vi "testpath3.vi"() -> (4 "Trajectory":T1[](array[typedef])=[{"t"=0.0, "velocity"=0.0, "acceleration"=1.5000000000000002, "pose"={"Translation2d"={"x"=3.048, "y"=7.32}, "Rotation2d"={"Theta"=0.0}}, "curvature"=0.0}, {"t"=0.26318841870669524, "velocity"=0.39478262806004294, "acceleration"=1.4999999999999998, "pose"={"Translation2d"={"x"=3.099949943360352, "y"=7.319652167962023}, "Rotation2d"={"Theta"=-0.019971918166744478}}, "curvature"=-0.7636115223795371}, {"t"=0.36948492482788675, "velocity"=0.5542273872418302, "acceleration"=0.9893258261872959, "pose"={"Translation2d"={"x"=3.1503355546365754, "y"=7.317348982771782}, "Rotation2d"={"Theta"=-0.07810185233815051}}, "curvature"=-1.5647606140766166}, {"t"=0.4117570606819468, "velocity"=0.5960483029703497, "acceleration"=-1.3031431956514083, "pose"={"Translation2d"={"x"=3.1745290416453305, "y"=7.3149482814664}, "Rotation2d"={"Theta"=-0.12154551781557867}}, "curvature"=-2.018124199473524}, {"t"=0.4532301831920973, "velocity"=0.5420028855688298, "acceleration"=-1.0963837092013367, "pose"={"Translation2d"={"x"=3.1978728847629, "y"=7.311485558945839}, "Rotation2d"={"Theta"=-0.1749375579100152}}, "curvature"=-2.516292087881445}, {"t"=0.4973792029848024, "velocity"=0.4935986194909005, "acceleration"=-0.8959940799444455, "pose"={"Translation2d"={"x"=3.2202513084556, "y"=7.3068161003781}, "Rotation2d"={"Theta"=-0.2385314594754074}}, "curvature"=-3.0550678047878725}, {"t"=0.5442304458911938, "velocity"=0.4516201832087346, "acceleration"=-0.6977078164312602, "pose"={"Translation2d"={"x"=3.241565206302116, "y"=7.3008160266614945}, "Rotation2d"={"Theta"=-0.31235747491337007}}, "curvature"=-3.6158302060928915}, {"t"=0.59371280358814, "velocity"=0.4170959554681277, "acceleration"=-0.5502702892987111, "pose"={"Translation2d"={"x"=3.2617314998738003, "y"=7.2933814930504015}, "Rotation2d"={"Theta"=-0.3960059769552128}}, "curvature"=-4.161606365084675}, {"t"=0.6194191597231453, "velocity"=0.40295051144090266, "acceleration"=-0.4537944570015777, "pose"={"Translation2d"={"x"=3.2713625579263197, "y"=7.289099133232461}, "Rotation2d"={"Theta"=-0.4412109262460302}}, "curvature"=-4.412233912146192}, {"t"=0.6456792669078144, "velocity"=0.39103382036023254, "acceleration"=-0.35872337751457745, "pose"={"Translation2d"={"x"=3.280682497614963, "y"=7.284427887781026}, "Rotation2d"={"Theta"=-0.48841072855155615}}, "curvature"=-4.637444890788882}, {"t"=0.672427300998411, "velocity"=0.3814386752293787, "acceleration"=-0.26515659471242126, "pose"={"Translation2d"={"x"=3.289685156510468, "y"=7.279360053903572}, "Rotation2d"={"Theta"=-0.5373459655625523}}, "curvature"=-4.829008235209974}, {"t"=0.6995828713909455, "velocity"=0.3742381966566208, "acceleration"=-0.17306381081986122, "pose"={"Translation2d"={"x"=3.2983652537231674, "y"=7.273889030697156}, "Rotation2d"={"Theta"=-0.5877071696426507}}, "curvature"=-4.979214634058512}, {"t"=0.7270527510074084, "velocity"=0.3694841546074329, "acceleration"=-0.08230445614380336, "pose"={"Translation2d"={"x"=3.306718369868, "y"=7.268009294105475}, "Rotation2d"={"Theta"=-0.6391410543429558}}, "curvature"=-5.081595546929804}, {"t"=0.7547338372219726, "velocity"=0.36720587786107345, "acceleration"=0.007327002008865816, "pose"={"Translation2d"={"x"=3.3147409270295203, "y"=7.26171637187592}, "Rotation2d"={"Theta"=-0.6912605824921104}}, "curvature"=-5.1315991090878725}, {"t"=0.7825171548337527, "velocity"=0.3674094462850279, "acceleration"=0.09603775765468281, "pose"={"Translation2d"={"x"=3.322430168726906, "y"=7.2550068185166285}, "Rotation2d"={"Theta"=-0.7436582689510873}}, "curvature"=-5.12710596463869}, {"t"=0.810292539234296, "velocity"=0.37007693192085295, "acceleration"=0.1839647992565535, "pose"={"Translation2d"={"x"=3.329784139878969, "y"=7.247878190253543}, "Rotation2d"={"Theta"=-0.7959215893197124}}, "curvature"=-5.06868621850621}, {"t"=0.8379535169277367, "velocity"=0.37516557812946677, "acceleration"=0.2711047475886817, "pose"={"Translation2d"={"x"=3.3368016667691625, "y"=7.240329019987463}, "Rotation2d"={"Theta"=-0.8476489989740198}}, "curvature"=-4.959545409978163}, {"t"=0.8654018650808298, "velocity"=0.38260695562723734, "acceleration"=0.35725561353969615, "pose"={"Translation2d"={"x"=3.3434823370105917, "y"=7.2323587922511035}, "Rotation2d"={"Theta"=-0.8984649589344123}}, "curvature"=-4.805170257332568}, {"t"=0.8925513920592509, "velocity"=0.3923062765452257, "acceleration"=0.4419796232654606, "pose"={"Translation2d"={"x"=3.349826479511024, "y"=7.223967918166147}, "Rotation2d"={"Theta"=-0.9480325468739267}}, "curvature"=-4.612744537302747}, {"t"=0.9193306197316901, "velocity"=0.40414214950323035, "acceleration"=0.5245940453086011, "pose"={"Translation2d"={"x"=3.355835144437894, "y"=7.2151577104002955}, "Rotation2d"={"Theta"=-0.9960626519615907}}, "curvature"=-4.39044385259067}, {"t"=0.945684227977588, "velocity"=0.4179670954614241, "acceleration"=0.6041935808611568, "pose"={"Translation2d"={"x"=3.361510083183318, "y"=7.205930358124334}, "Rotation2d"={"Theta"=-1.0423192986977439}}, "curvature"=-4.146726130102364}, {"t"=0.9715732984686114, "velocity"=0.4336091056665624, "acceleration"=0.7153350615387603, "pose"={"Translation2d"={"x"=3.3668537283290987, "y"=7.1962889019691785}, "Rotation2d"={"Theta"=-1.0866211858450743}}, "curvature"=-3.889714967048319}, {"t"=1.0218188627011469, "velocity"=0.46955151944889295, "acceleration"=0.8424284702084108, "pose"={"Translation2d"={"x"=3.376560153887442, "y"=7.17577994758794}, "Rotation2d"={"Theta"=-1.1688959585687513}}, "curvature"=-3.364030064250997}, {"t"=1.0701152351915793, "velocity"=0.5102377586426234, "acceleration"=0.9380799882762356, "pose"={"Translation2d"={"x"=3.3849867442314645, "y"=7.153671249874651}, "Rotation2d"={"Theta"=-1.2424085833564584}}, "curvature"=-2.8583316258579563}, {"t"=1.116586221907962, "velocity"=0.553831261316713, "acceleration"=0.9976984170949652, "pose"={"Translation2d"={"x"=3.392175439275308, "y"=7.130015232061024}, "Rotation2d"={"Theta"=-1.307257225938115}}, "curvature"=-2.398952122349185}, {"t"=1.1614418998127427, "velocity"=0.5985837001600341, "acceleration"=1.0215095892207162, "pose"={"Translation2d"={"x"=3.3981771546090056, "y"=7.1048755366181675}, "Rotation2d"={"Theta"=-1.363907802949199}}, "curvature"=-1.9969630345874718}, {"t"=1.2049234360760661, "velocity"=0.6430005064070674, "acceleration"=1.0141956822707063, "pose"={"Translation2d"={"x"=3.4030511403787758, "y"=7.07832622388235}, "Rotation2d"={"Theta"=-1.4130182829288858}}, "curvature"=-1.6533172386850903}, {"t"=1.2472651193286828, "velocity"=0.6859432587419452, "acceleration"=0.9602009106383614, "pose"={"Translation2d"={"x"=3.406864340167318, "y"=7.050450970680747}, "Rotation2d"={"Theta"=-1.4553132146872148}}, "curvature"=-1.3633891597444852}, {"t"=1.3293491957534012, "velocity"=0.7647604636738685, "acceleration"=0.8586816816302829, "pose"={"Translation2d"={"x"=3.4116107765956682, "y"=6.99110062439801}, "Rotation2d"={"Theta"=-1.5222489468742204}}, "curvature"=-0.9159774788659977}, {"t"=1.4087890285949973, "velocity"=0.8329739929267188, "acceleration"=0.7675452912761603, "pose"={"Translation2d"={"x"=3.413081518736379, "y"=6.927655789984416}, "Rotation2d"={"Theta"=-1.5696286047023655}}, "curvature"=-0.5971075544889111}, {"t"=1.4860126079520202, "velocity"=0.8922465876376926, "acceleration"=0.7215507468236929, "pose"={"Translation2d"={"x"=3.41202368475422, "y"=6.861050335557494}, "Rotation2d"={"Theta"=-1.6010972924732694}}, "curvature"=-0.35962182913643914}, {"t"=1.5608683710367142, "velocity"=0.946258819395511, "acceleration"=0.7477618287923464, "pose"={"Translation2d"={"x"=3.4092459403057958, "y"=6.792295061162074}, "Rotation2d"={"Theta"=-1.6190734369903932}}, "curvature"=-0.16912085734671656}, {"t"=1.6327377531517113, "velocity"=0.9999999999999973, "acceleration"=-0.7477618287922758, "pose"={"Translation2d"={"x"=3.405597982708933, "y"=6.7224520547945215}, "Rotation2d"={"Theta"=-1.6249193382438716}}, "curvature"=-7.901475617054195e-15}, {"t"=1.7046071352667083, "velocity"=0.9462588193955163, "acceleration"=-0.7215507468237041, "pose"={"Translation2d"={"x"=3.40195002511207, "y"=6.652609048426969}, "Rotation2d"={"Theta"=-1.6190734369903943}}, "curvature"=0.16912085734669927}, {"t"=1.779462898351402, "velocity"=0.8922465876376973, "acceleration"=-0.7675452912761632, "pose"={"Translation2d"={"x"=3.3991722806636457, "y"=6.583853774031549}, "Rotation2d"={"Theta"=-1.6010972924732707}}, "curvature"=0.3596218291364221}, {"t"=1.8566864777084247, "velocity"=0.8329739929267235, "acceleration"=-0.8586816816302913, "pose"={"Translation2d"={"x"=3.398114446681486, "y"=6.517248319604627}, "Rotation2d"={"Theta"=-1.5696286047023693}}, "curvature"=0.5971075544888911}, {"t"=1.9361263105500202, "velocity"=0.764760463673873, "acceleration"=-0.9602009106384005, "pose"={"Translation2d"={"x"=3.399585188822197, "y"=6.453803485191033}, "Rotation2d"={"Theta"=-1.5222489468742246}}, "curvature"=0.9159774788659754}, {"t"=2.0182103869747365, "velocity"=0.6859432587419481, "acceleration"=-1.0141956822706626, "pose"={"Translation2d"={"x"=3.4043316252505473, "y"=6.394453138908297}, "Rotation2d"={"Theta"=-1.4553132146872205}}, "curvature"=1.3633891597444665}, {"t"=2.060552070227354, "velocity"=0.6430005064070712, "acceleration"=-1.0215095892206796, "pose"={"Translation2d"={"x"=3.408144825039089, "y"=6.366577885706693}, "Rotation2d"={"Theta"=-1.4130182829288918}}, "curvature"=1.6533172386850632}, {"t"=2.104033606490679, "velocity"=0.5985837001600383, "acceleration"=-0.9976984170950692, "pose"={"Translation2d"={"x"=3.4130188108088593, "y"=6.3400285729708745}, "Rotation2d"={"Theta"=-1.3639078029492069}}, "curvature"=1.9969630345874378}, {"t"=2.148889284395456, "velocity"=0.5538312613167158, "acceleration"=-0.9380799882762958, "pose"={"Translation2d"={"x"=3.4190205261425564, "y"=6.31488887752802}, "Rotation2d"={"Theta"=-1.307257225938124}}, "curvature"=2.3989521223491583}, {"t"=2.1953602711118387, "velocity"=0.5102377586426238, "acceleration"=-0.8424284702084165, "pose"={"Translation2d"={"x"=3.4262092211863995, "y"=6.291232859714393}, "Rotation2d"={"Theta"=-1.2424085833564666}}, "curvature"=2.8583316258579528}, {"t"=2.2436566436022707, "velocity"=0.4695515194488933, "acceleration"=-0.7153350615388038, "pose"={"Translation2d"={"x"=3.4346358115304216, "y"=6.269124162001104}, "Rotation2d"={"Theta"=-1.1688959585687604}}, "curvature"=3.364030064250993}, {"t"=2.2939022078348064, "velocity"=0.4336091056665604, "acceleration"=-0.6041935808611378, "pose"={"Translation2d"={"x"=3.444342237088765, "y"=6.248615207619865}, "Rotation2d"={"Theta"=-1.0866211858450845}}, "curvature"=3.889714967048351}, {"t"=2.3197912783258308, "velocity"=0.4179670954614221, "acceleration"=-0.5245940453086523, "pose"={"Translation2d"={"x"=3.4496858822345446, "y"=6.238973751464709}, "Rotation2d"={"Theta"=-1.0423192986977563}}, "curvature"=4.146726130102398}, {"t"=2.3461448865717274, "velocity"=0.40414214950322763, "acceleration"=-0.4419796232654363, "pose"={"Translation2d"={"x"=3.455360820979969, "y"=6.229746399188748}, "Rotation2d"={"Theta"=-0.9960626519616042}}, "curvature"=4.390443852590719}, {"t"=2.3729241142441673, "velocity"=0.3923062765452232, "acceleration"=-0.35725561353967616, "pose"={"Translation2d"={"x"=3.4613694859068396, "y"=6.220936191422897}, "Rotation2d"={"Theta"=-0.9480325468739386}}, "curvature"=4.612744537302796}, {"t"=2.4000736412225905, "velocity"=0.3826069556272347, "acceleration"=-0.27110474758883285, "pose"={"Translation2d"={"x"=3.467713628407272, "y"=6.2125453173379395}, "Rotation2d"={"Theta"=-0.8984649589344248}}, "curvature"=4.805170257332622}, {"t"=2.42752198937568, "velocity"=0.37516557812946094, "acceleration"=-0.18396479925663856, "pose"={"Translation2d"={"x"=3.4743942986486998, "y"=6.2045750896015806}, "Rotation2d"={"Theta"=-0.8476489989740319}}, "curvature"=4.959545409978286}, {"t"=2.45518296706912, "velocity"=0.3700769319208449, "acceleration"=-0.09603775765469771, "pose"={"Translation2d"={"x"=3.4814118255388937, "y"=6.197025919335502}, "Rotation2d"={"Theta"=-0.7959215893197208}}, "curvature"=5.068686218506383}, {"t"=2.482958351469662, "velocity"=0.3674094462850196, "acceleration"=-0.007327002008889338, "pose"={"Translation2d"={"x"=3.4887657966909558, "y"=6.189897291072416}, "Rotation2d"={"Theta"=-0.743658268951097}}, "curvature"=5.127105964638875}, {"t"=2.510741669081451, "velocity"=0.3672058778610644, "acceleration"=0.0823044561438033, "pose"={"Translation2d"={"x"=3.4964550383883424, "y"=6.183187737713124}, "Rotation2d"={"Theta"=-0.6912605824921165}}, "curvature"=5.1315991090880715}, {"t"=2.538422755296015, "velocity"=0.3694841546074238, "acceleration"=0.173063810819882, "pose"={"Translation2d"={"x"=3.5044775955498615, "y"=6.176894815483568}, "Rotation2d"={"Theta"=-0.6391410543429624}}, "curvature"=5.081595546930003}, {"t"=2.565892634912475, "velocity"=0.37423819665661173, "acceleration"=0.2651565947124028, "pose"={"Translation2d"={"x"=3.5128307116946935, "y"=6.171015078891888}, "Rotation2d"={"Theta"=-0.5877071696426573}}, "curvature"=4.979214634058704}, {"t"=2.5930482053050126, "velocity"=0.38143867522937003, "acceleration"=0.35872337751447186, "pose"={"Translation2d"={"x"=3.521510808907394, "y"=6.165544055685473}, "Rotation2d"={"Theta"=-0.5373459655625578}}, "curvature"=4.82900823521015}, {"t"=2.619796239395607, "velocity"=0.3910338203602203, "acceleration"=0.45379445700158316, "pose"={"Translation2d"={"x"=3.5305134678028973, "y"=6.160476221808018}, "Rotation2d"={"Theta"=-0.48841072855156026}}, "curvature"=4.637444890789121}, {"t"=2.6460563465802767, "velocity"=0.40295051144089095, "acceleration"=0.5502702892986385, "pose"={"Translation2d"={"x"=3.539833407491541, "y"=6.155804976356584}, "Rotation2d"={"Theta"=-0.4412109262460335}}, "curvature"=4.412233912146407}, {"t"=2.671762702715285, "velocity"=0.4170959554681157, "acceleration"=0.697707816431294, "pose"={"Translation2d"={"x"=3.5494644655440615, "y"=6.151522616538643}, "Rotation2d"={"Theta"=-0.3960059769552175}}, "curvature"=4.161606365084881}, {"t"=2.721245060412225, "velocity"=0.45162018320872005, "acceleration"=0.8959940799443867, "pose"={"Translation2d"={"x"=3.569630759115743, "y"=6.144088082927551}, "Rotation2d"={"Theta"=-0.31235747491337135}}, "curvature"=3.615830206093104}, {"t"=2.7680963033186217, "velocity"=0.4935986194908878, "acceleration"=1.096383709201355, "pose"={"Translation2d"={"x"=3.59094465696226, "y"=6.138088009210944}, "Rotation2d"={"Theta"=-0.2385314594754091}}, "curvature"=3.055067804788028}, {"t"=2.812245323111325, "velocity"=0.542002885568816, "acceleration"=1.3031431956514576, "pose"={"Translation2d"={"x"=3.6133230806549586, "y"=6.1334185506432055}, "Rotation2d"={"Theta"=-0.17493755791001384}}, "curvature"=2.516292087881585}, {"t"=2.853718445621474, "velocity"=0.5960483029703362, "acceleration"=1.4999999999999967, "pose"={"Translation2d"={"x"=3.636666923772527, "y"=6.129955828122645}, "Rotation2d"={"Theta"=-0.12154551781557543}}, "curvature"=2.0181241994736374}, {"t"=2.892604873611095, "velocity"=0.6543779449547675, "acceleration"=1.4999999999999962, "pose"={"Translation2d"={"x"=3.660860410781282, "y"=6.127555126817265}, "Rotation2d"={"Theta"=-0.0781018523381434}}, "curvature"=1.5647606140767099}, {"t"=2.963863246576663, "velocity"=0.7612655044031196, "acceleration"=1.0405196335401754, "pose"={"Translation2d"={"x"=3.711246022057505, "y"=6.125251941627026}, "Rotation2d"={"Theta"=-0.01997191816673276}}, "curvature"=0.763611522379592}, {"t"=3.029189820400926, "velocity"=0.8292390870591767, "acceleration"=-1.5, "pose"={"Translation2d"={"x"=3.7631959654178546, "y"=6.124904109589046}, "Rotation2d"={"Theta"=8.502859727842416e-15}}, "curvature"=1.0175126690166933e-14}, {"t"=3.0957507797886894, "velocity"=0.7293976479775318, "acceleration"=-1.5, "pose"={"Translation2d"={"x"=3.8150667797484186, "y"=6.125280265127143}, "Rotation2d"={"Theta"=0.02169629189301651}}, "curvature"=0.8370645436394706}, {"t"=3.169839919062551, "velocity"=0.6182639390667396, "acceleration"=-1.499999999999999, "pose"={"Translation2d"={"x"=3.8649281521524923, "y"=6.127770995623446}, "Rotation2d"={"Theta"=0.08595677451778284}}, "curvature"=1.782517383837334}, {"t"=3.2103029683127233, "velocity"=0.5575693651914811, "acceleration"=-1.4457439691216696, "pose"={"Translation2d"={"x"=3.8885749615894682, "y"=6.130367182842418}, "Rotation2d"={"Theta"=0.1350468581629947}}, "curvature"=2.362904642794918}, {"t"=3.25375724435825, "velocity"=0.49474560766611264, "acceleration"=-1.2078309552388122, "pose"={"Translation2d"={"x"=3.911130012707782, "y"=6.1341118702512905}, "Rotation2d"={"Theta"=0.1965838508185219}}, "curvature"=3.041081500714643}, {"t"=3.3007238350701016, "velocity"=0.43801790554230635, "acceleration"=-1.02600305040188, "pose"={"Translation2d"={"x"=3.932444367068773, "y"=6.139161556618315}, "Rotation2d"={"Theta"=0.2715148453026895}}, "curvature"=3.8205907799824077}, {"t"=3.3256552410396116, "velocity"=0.41243820696678135, "acceleration"=-0.9042303566046068, "pose"={"Translation2d"={"x"=3.9425956051051148, "y"=6.142218495388199}, "Rotation2d"={"Theta"=0.31423417016703553}}, "curvature"=4.242233471704546}, {"t"=3.351554605820681, "velocity"=0.3890192151149621, "acceleration"=-0.7827247383890393, "pose"={"Translation2d"={"x"=3.9523904547627575, "y"=6.14565020835563}, "Rotation2d"={"Theta"=0.3605071157677527}}, "curvature"=4.676881947505758}, {"t"=3.3784244404446717, "velocity"=0.36798753083834224, "acceleration"=-0.662602475512602, "pose"={"Translation2d"={"x"=3.9618161739669553, "y"=6.149470062822817}, "Rotation2d"={"Theta"=0.4102979234949962}}, "curvature"=5.114373635616514}, {"t"=3.4062447276670778, "velocity"=0.3495537396553043, "acceleration"=-0.544869386173178, "pose"={"Translation2d"={"x"=3.970861253571306, "y"=6.153690126148347}, "Rotation2d"={"Theta"=0.4634900930941465}}, "curvature"=5.541117727082771}, {"t"=3.434967334665074, "velocity"=0.33390367041101254, "acceleration"=-0.43022831997720556, "pose"={"Translation2d"={"x"=3.9795153917065753, "y"=6.158321192829343}, "Rotation2d"={"Theta"=0.5198699448216426}}, "curvature"=5.940400917104992}, {"t"=3.4645117522286055, "velocity"=0.32119282527794935, "acceleration"=-0.31896297108270455, "pose"={"Translation2d"={"x"=3.987769468129517, "y"=6.163372811583624}, "Rotation2d"={"Theta"=0.579114543882686}}, "curvature"=6.293329886337889}, {"t"=3.494763207006263, "velocity"=0.31154373138249364, "acceleration"=-0.21090669660756495, "pose"={"Translation2d"={"x"=3.995615518571693, "y"=6.168853312431866}, "Rotation2d"={"Theta"=0.6407871610915412}}, "curvature"=6.580475104760627}, {"t"=3.5255740996295852, "velocity"=0.30504550779977835, "acceleration"=-0.10549365407667427, "pose"={"Translation2d"={"x"=4.003046709088297, "y"=6.174769833779754}, "Rotation2d"={"Theta"=0.704343118936269}}, "curvature"=6.784090638880426}, {"t"=3.556769319971538, "velocity"=0.30175461001617876, "acceleration"=-0.00187984418221485, "pose"={"Translation2d"={"x"=4.010057310406972, "y"=6.181128349500149}, "Rotation2d"={"Theta"=0.7691476236098183}}, "curvature"=6.89055291686925}, {"t"=3.588155300244517, "velocity"=0.3016956092637595, "acceleration"=0.10088508839139915, "pose"={"Translation2d"={"x"=4.016642672276634, "y"=6.187933696015241}, "Rotation2d"={"Theta"=0.8345050811793373}}, "curvature"=6.892482815756199}, {"t"=3.619531844801653, "velocity"=0.30486103473482284, "acceleration"=0.2036584602787223, "pose"={"Translation2d"={"x"=4.022799197816295, "y"=6.195189599378709}, "Rotation2d"={"Theta"=0.8996969187800614}}, "curvature"=6.789997630017758}, {"t"=3.6507050870217803, "velocity"=0.3112097292472697, "acceleration"=0.3070031169576213, "pose"={"Translation2d"={"x"=4.028524317863877, "y"=6.202898702357883}, "Rotation2d"={"Theta"=0.964022866726053}}, "curvature"=6.590733441928565}, {"t"=3.6814996282233716, "velocity"=0.32066374938143816, "acceleration"=0.4110109916433966, "pose"={"Translation2d"={"x"=4.033816465325044, "y"=6.211062591515899}, "Rotation2d"={"Theta"=1.0268397706121166}}, "curvature"=6.308626742522132}, {"t"=3.711768130749851, "velocity"=0.3331044366204071, "acceleration"=0.5151787076413319, "pose"={"Translation2d"={"x"=4.038675049522012, "y"=6.219681824293856}, "Rotation2d"={"Theta"=1.087592646120109}}, "curvature"=5.96179886550171}, {"t"=3.7413972791782246, "velocity"=0.34836874301624976, "acceleration"=0.6183591380506606, "pose"={"Translation2d"={"x"=4.043100430542376, "y"=6.228755956092982}, "Rotation2d"={"Theta"=1.1458346067318108}}, "curvature"=5.570095425836476}, {"t"=3.77030984430284, "velocity"=0.3662470918655407, "acceleration"=0.7188046863919453, "pose"={"Translation2d"={"x"=4.047093893587934, "y"=6.238283567356788}, "Rotation2d"={"Theta"=1.201234763455285}}, "curvature"=5.152828512098055}, {"t"=3.798463311036893, "velocity"=0.38648393569215755, "acceleration"=0.8143044023369251, "pose"={"Translation2d"={"x"=4.050657623323499, "y"=6.248262290653226}, "Rotation2d"={"Theta"=1.2535754049779992}}, "curvature"=4.727095765043343}, {"t"=3.8258459843159427, "velocity"=0.40878176709104125, "acceleration"=0.9023998533373291, "pose"={"Translation2d"={"x"=4.053794678225729, "y"=6.25868883775685}, "Rotation2d"={"Theta"=1.3027411728436462}}, "curvature"=4.30681494355726}, {"t"=3.8524716267039065, "velocity"=0.43280874287695215, "acceleration"=0.9806482024487537, "pose"={"Translation2d"={"x"=4.056508964931945, "y"=6.269559026730973}, "Rotation2d"={"Theta"=1.3487034150678558}}, "curvature"=3.9024146353943783}, {"t"=3.8783735764649694, "velocity"=0.4582094433500563, "acceleration"=1.0737791801596355, "pose"={"Translation2d"={"x"=4.05880521258895, "y"=6.280867809009828}, "Rotation2d"={"Theta"=1.3915026250306526}}, "curvature"=3.5210103734247618}, {"t"=3.9281613757118374, "velocity"=0.511670545607311, "acceleration"=1.1493157053378875, "pose"={"Translation2d"={"x"=4.0621664659828935, "y"=6.304776788566211}, "Rotation2d"={"Theta"=1.468017807371216}}, "curvature"=2.841989124902466}, {"t"=3.9757359053738783, "velocity"=0.5663486997219579, "acceleration"=1.1670145631573443, "pose"={"Translation2d"={"x"=4.06393174702687, "y"=6.330359084440269}, "Rotation2d"={"Theta"=1.5333858309580786}}, "curvature"=2.2801144879387643}, {"t"=4.0215762991318815, "velocity"=0.6198451068184146, "acceleration"=1.1006743364612166, "pose"={"Translation2d"={"x"=4.06416588281649, "y"=6.357545871839132}, "Rotation2d"={"Theta"=1.588929308641928}}, "curvature"=1.8263218570407036}, {"t"=4.109815546037458, "velocity"=0.7169677813560476, "acceleration"=0.9318625883402352, "pose"={"Translation2d"={"x"=4.0603526943702315, "y"=6.4164021577786094}, "Rotation2d"={"Theta"=1.675700032982171}}, "curvature"=1.1755365710921948}, {"t"=4.195430482937836, "velocity"=0.79674913805662, "acceleration"=0.7523290288742276, "pose"={"Translation2d"={"x"=4.05144469510141, "y"=6.480585323804046}, "Rotation2d"={"Theta"=1.737246271947655}}, "curvature"=0.7596450332214446}, {"t"=4.279755261190648, "velocity"=0.8601891165895926, "acceleration"=0.6143533949739849, "pose"={"Translation2d"={"x"=4.038291441473745, "y"=6.549196386681844}, "Rotation2d"={"Theta"=1.7799721406425593}}, "curvature"=0.4840017650067866}, {"t"=4.363161607728101, "velocity"=0.911430088747253, "acceleration"=0.5350736721146327, "pose"={"Translation2d"={"x"=4.021847985150234, "y"=6.621225434656013}, "Rotation2d"={"Theta"=1.8081197219754728}}, "curvature"=0.2893761649681477}, {"t"=4.445300886137392, "velocity"=0.9553806540705587, "acceleration"=0.5216342862430297, "pose"={"Translation2d"={"x"=4.003148606186002, "y"=6.69557935957876}, "Rotation2d"={"Theta"=1.8243223962345434}}, "curvature"=0.1390742305568728}, {"t"=4.525300854255131, "velocity"=0.9971113803391205, "acceleration"=-0.4536998073169741, "pose"={"Translation2d"={"x"=3.9832805462211565, "y"=6.771109589041096}, "Rotation2d"={"Theta"=1.8300183745307899}}, "curvature"=0.00862673780876401}, {"t"=4.605089090371286, "velocity"=0.9609114729870597, "acceleration"=-0.5365543906927763, "pose"={"Translation2d"={"x"=3.9633577416736303, "y"=6.846639818503432}, "Rotation2d"={"Theta"=1.8256865496810237}}, "curvature"=-0.12113393775215417}, {"t"=4.686782126161709, "velocity"=0.9170787159446863, "acceleration"=-0.6130323265414291, "pose"={"Translation2d"={"x"=3.9444945569320353, "y"=6.9209937434261795}, "Rotation2d"={"Theta"=1.8109242098580547}}, "curvature"=-0.2692522327535906}, {"t"=4.769709532055165, "velocity"=0.8662415353757755, "acceleration"=-0.7505687846392907, "pose"={"Translation2d"={"x"=3.927779517548515, "y"=6.993022791400348}, "Rotation2d"={"Theta"=1.7843770627090099}}, "curvature"=-0.45981398932552625}, {"t"=4.853480716504348, "velocity"=0.8033654992759588, "acceleration"=-0.9338371634647636, "pose"={"Translation2d"={"x"=3.9142490434315893, "y"=7.061633854278146}, "Rotation2d"={"Theta"=1.7435098835081497}}, "curvature"=-0.7288639189517633}, {"t"=4.938416516388425, "velocity"=0.7240492928356015, "acceleration"=-1.1128693674812653, "pose"={"Translation2d"={"x"=3.9048611820390096, "y"=7.125817020303582}, "Rotation2d"={"Theta"=1.6841931776688028}}, "curvature"=-1.1349148706994323}, {"t"=5.025798137602182, "velocity"=0.6268049633059594, "acceleration"=-1.1909833664174907, "pose"={"Translation2d"={"x"=3.900469341570604, "y"=7.184673306243059}, "Rotation2d"={"Theta"=1.600125971053358}}, "curvature"=-1.7729779784640636}, {"t"=5.0711237586504465, "velocity"=0.5728229025649334, "acceleration"=-1.1815955171284798, "pose"={"Translation2d"={"x"=3.900378542851255, "y"=7.211860093641923}, "Rotation2d"={"Theta"=1.5461204056689204}}, "curvature"=-2.220687744773954}, {"t"=5.118131359885848, "velocity"=0.5172789316742191, "acceleration"=-1.1128857445929383, "pose"={"Translation2d"={"x"=3.901796024161135, "y"=7.237442389515981}, "Rotation2d"={"Theta"=1.4823867426308168}}, "curvature"=-2.7788901065523715}, {"t"=5.167314501619449, "velocity"=0.46254371436460084, "acceleration"=-0.9853196967791875, "pose"={"Translation2d"={"x"=3.9047873347963726, "y"=7.261351369072363}, "Rotation2d"={"Theta"=1.4075396162447975}}, "curvature"=-3.4601129169826157}, {"t"=5.219155935278846, "velocity"=0.41146332867072566, "acceleration"=-0.8579361355402367, "pose"={"Translation2d"={"x"=3.9094065590731395, "y"=7.283530340325342}, "Rotation2d"={"Theta"=1.3203628208481204}}, "curvature"=-4.259339937185443}, {"t"=5.24624506210542, "velocity"=0.3882225878859752, "acceleration"=-0.7617675977105636, "pose"={"Translation2d"={"x"=3.912340203217406, "y"=7.293956887428966}, "Rotation2d"={"Theta"=1.2719031149667976}}, "curvature"=-4.6925893076690235}, {"t"=5.274125426904337, "velocity"=0.36698422936981007, "acceleration"=-0.6600149113578105, "pose"={"Translation2d"={"x"=3.915695495489917, "y"=7.303935610725403}, "Rotation2d"={"Theta"=1.2201732587521121}}, "curvature"=-5.136496983697817}, {"t"=5.302795200406767, "velocity"=0.3480617513529555, "acceleration"=-0.5551081415780252, "pose"={"Translation2d"={"x"=3.919475606375281, "y"=7.31346322198921}, "Rotation2d"={"Theta"=1.1652564437436912}}, "curvature"=-5.577634725546802}, {"t"=5.33222209949546, "velocity"=0.33172664008742736, "acceleration"=-0.449032030653943, "pose"={"Translation2d"={"x"=3.923682835889786, "y"=7.322537353788336}, "Rotation2d"={"Theta"=1.107337414512981}}, "curvature"=-5.998928803965122}, {"t"=5.36233855927511, "velocity"=0.31820338499646317, "acceleration"=-0.3431550910056521, "pose"={"Translation2d"={"x"=3.9283185879302205, "y"=7.331156586566293}, "Rotation2d"={"Theta"=1.046716215748132}}, "curvature"=-6.380430087945608}, {"t"=5.393039206588993, "velocity"=0.3076683015735352, "acceleration"=-0.23815674690757505, "pose"={"Translation2d"={"x"=3.9333833446226927, "y"=7.339320475724309}, "Rotation2d"={"Theta"=0.9838145805699728}}, "curvature"=-6.700872755577214}, {"t"=5.424181717947586, "velocity"=0.3002515023778406, "acceleration"=-0.13405431784570007, "pose"={"Translation2d"={"x"=3.9388766406714555, "y"=7.347029578703482}, "Rotation2d"={"Theta"=0.9191717247022226}}, "curvature"=-6.9399556399395745}, {"t"=5.4555917701745775, "velocity"=0.2960408492530534, "acceleration"=-0.030315741458309037, "pose"={"Translation2d"={"x"=3.944797037707727, "y"=7.35428548206695}, "Rotation2d"={"Theta"=0.8534274890518816}}, "curvature"=-7.081018454188822}, {"t"=5.487072081656566, "velocity"=0.2950865002691384, "acceleration"=0.07396602536212296, "pose"={"Translation2d"={"x"=3.951142098638508, "y"=7.361090828582042}, "Rotation2d"={"Theta"=0.7872929428384307}}, "curvature"=-7.113550107943131}, {"t"=5.518414645078499, "velocity"=0.29740478511011903, "acceleration"=0.17986505233896102, "pose"={"Translation2d"={"x"=3.957908361995406, "y"=7.367449344302436}, "Rotation2d"={"Theta"=0.7215112626164027}}, "curvature"=-7.034887306172089}, {"t"=5.549414452573213, "velocity"=0.3029805671076536, "acceleration"=0.288409203225415, "pose"={"Translation2d"={"x"=3.9650913162834547, "y"=7.373365865650326}, "Rotation2d"={"Theta"=0.656814093888202}}, "curvature"=-6.850622256624144}, {"t"=5.579882613827221, "velocity"=0.3117678652186653, "acceleration"=0.4003883683441281, "pose"={"Translation2d"={"x"=3.9726853743299397, "y"=7.378846366498566}, "Rotation2d"={"Theta"=0.5938797909916396}}, "curvature"=-6.573603519065585}, {"t"=5.609656930959911, "velocity"=0.3236891554739839, "acceleration"=0.5162087737657857, "pose"={"Translation2d"={"x"=3.9806838476332143, "y"=7.383897985252849}, "Rotation2d"={"Theta"=0.5332994383480224}}, "curvature"=-6.221829571535764}, {"t"=5.638608652780793, "velocity"=0.33863428829354947, "acceleration"=0.6358147702330265, "pose"={"Translation2d"={"x"=3.9890789207115187, "y"=7.388529051933843}, "Rotation2d"={"Theta"=0.4755545834394751}}, "curvature"=-5.815815946306666}, {"t"=5.666645024556614, "velocity"=0.35646022757236073, "acceleration"=0.7586938982961912, "pose"={"Translation2d"={"x"=3.9978616254518116, "y"=7.392749115259375}, "Rotation2d"={"Theta"=0.4210079262946777}}, "curvature"=-5.376061416802838}, {"t"=5.693708067282841, "velocity"=0.3769927929580783, "acceleration"=0.8839721704593035, "pose"={"Translation2d"={"x"=4.007021815458583, "y"=7.3965689697265615}, "Rotation2d"={"Theta"=0.36990573115036535}}, "curvature"=-4.9210744088842135}, {"t"=5.719770547259522, "velocity"=0.40003129995061737, "acceleration"=1.010595158151202, "pose"={"Translation2d"={"x"=4.016548140402675, "y"=7.4000006826939915}, "Rotation2d"={"Theta"=0.32238910169973845}}, "curvature"=-4.466162591352536}, {"t"=5.744830274468121, "velocity"=0.4253565389322175, "acceleration"=1.2018608892153573, "pose"={"Translation2d"={"x"=4.026428020370103, "y"=7.403057621463877}, "Rotation2d"={"Theta"=0.27851067991033035}}, "curvature"=-4.022955833028221}, {"t"=5.7919336221573525, "velocity"=0.48196821027101827, "acceleration"=1.455458010218352, "pose"={"Translation2d"={"x"=4.047191823887849, "y"=7.4081073078309005}, "Rotation2d"={"Theta"=0.2015502334025534}}, "curvature"=-3.200648092862073}, {"t"=5.835376810367199, "velocity"=0.5451979465404633, "acceleration"=1.500000000000012, "pose"={"Translation2d"={"x"=4.069187020258681, "y"=7.411851995239773}, "Rotation2d"={"Theta"=0.1383803127731085}}, "curvature"=-2.4840945065364326}, {"t"=5.875734741636085, "velocity"=0.6057348434437911, "acceleration"=1.4999999999999953, "pose"={"Translation2d"={"x"=4.0922660886968085, "y"=7.414448182458744}, "Rotation2d"={"Theta"=0.0880295645890188}}, "curvature"=-1.8713804756786312}, {"t"=5.9495120585780255, "velocity"=0.7164008188567023, "acceleration"=1.5000000000000033, "pose"={"Translation2d"={"x"=4.140974258442265, "y"=7.416938912955046}, "Rotation2d"={"Theta"=0.02220021162873243}}, "curvature"=-0.8766770741906679}, {"t"=6.015703779688769, "velocity"=0.815688400522817, "acceleration"=-1.411158753722337, "pose"={"Translation2d"={"x"=4.191678674351594, "y"=7.417315068493148}, "Rotation2d"={"Theta"=-4.348736071993605e-15}}, "curvature"=4.6297649204425944e-29}, {"t"=6.081632420221635, "velocity"=0.72265262231385, "acceleration"=-1.5, "pose"={"Translation2d"={"x"=4.242387725084967, "y"=7.416949816014125}, "Rotation2d"={"Theta"=-0.021551071408703826}}, "curvature"=-0.8506112665210034}, {"t"=6.154699751119267, "velocity"=0.6130516259674026, "acceleration"=-1.500000000000001, "pose"={"Translation2d"={"x"=4.291125926643832, "y"=7.414531280604673}, "Rotation2d"={"Theta"=-0.08540110372174131}}, "curvature"=-1.8127044897775162}, {"t"=6.194563863764197, "velocity"=0.5532554570000089, "acceleration"=-1.4742082201926978, "pose"={"Translation2d"={"x"=4.314235733500783, "y"=7.412010345189149}, "Rotation2d"={"Theta"=-0.13420095994761355}}, "curvature"=-2.404548044357114}, {"t"=6.237379696389456, "velocity"=0.49013600458945655, "acceleration"=-1.2297545468345767, "pose"={"Translation2d"={"x"=4.336274624928279, "y"=7.408374199444301}, "Rotation2d"={"Theta"=-0.19540776415030497}}, "curvature"=-3.0976878160366175}, {"t"=6.283717050284497, "velocity"=0.43315243294874783, "acceleration"=-1.0438639863352206, "pose"={"Translation2d"={"x"=4.357096446235751, "y"=7.403470880798062}, "Rotation2d"={"Theta"=-0.2699944269844921}}, "curvature"=-3.896955421473778}, {"t"=6.3083408507292775, "velocity"=0.4074485344577359, "acceleration"=-0.9198414890264246, "pose"={"Translation2d"={"x"=4.367011030837094, "y"=7.400502548949043}, "Rotation2d"={"Theta"=-0.31254883046411347}}, "curvature"=-4.330651393103863}, {"t"=6.333939580128287, "velocity"=0.3839017610901667, "acceleration"=-0.7964221481695049, "pose"={"Translation2d"={"x"=4.376575985710204, "y"=7.397170305922697}, "Rotation2d"={"Theta"=-0.35867079037891914}}, "curvature"=-4.778920126845849}, {"t"=6.360517915374173, "velocity"=0.3627341862388689, "acceleration"=-0.6747263638224956, "pose"={"Translation2d"={"x"=4.385778799803259, "y"=7.393461171874849}, "Rotation2d"={"Theta"=-0.40833284223567334}}, "curvature"=-5.231570018449862}, {"t"=6.388058201331983, "velocity"=0.3441520292359239, "acceleration"=-0.5557590542485462, "pose"={"Translation2d"={"x"=4.394608170484017, "y"=7.389363429225421}, "Rotation2d"={"Theta"=-0.4614276486470032}}, "curvature"=-5.674828660300538}, {"t"=6.416514699519203, "velocity"=0.32833707271616924, "acceleration"=-0.44021373956923865, "pose"={"Translation2d"={"x"=4.403053978410674, "y"=7.384866596361266}, "Rotation2d"={"Theta"=-0.5177510355035748}}, "curvature"=-6.091599816339996}, {"t"=6.445809083367991, "velocity"=0.31544128245371733, "acceleration"=-0.32835366155801143, "pose"={"Translation2d"={"x"=4.411107262402737, "y"=7.379961401338992}, "Rotation2d"={"Theta"=-0.5769891409471082}}, "curvature"=-6.46237394112836}, {"t"=6.4758282443560695, "velocity"=0.3055843810263824, "acceleration"=-0.2199782815004123, "pose"={"Translation2d"={"x"=4.418760194311893, "y"=7.374639755587801}, "Rotation2d"={"Theta"=-0.6387129060337345}}, "curvature"=-6.766876284911729}, {"t"=6.506425405606849, "velocity"=0.29885367007564506, "acceleration"=-0.11447227589115234, "pose"={"Translation2d"={"x"=4.426006053892873, "y"=7.368894727612315}, "Rotation2d"={"Theta"=-0.7023828897284222}}, "curvature"=-6.986344232749775}, {"t"=6.537425160306578, "velocity"=0.29530505760309966, "acceleration"=-0.010924686245635714, "pose"={"Translation2d"={"x"=4.432839203674328, "y"=7.3627205166954095}, "Rotation2d"={"Theta"=-0.767366208906101}}, "curvature"=-7.106081407060201}, {"t"=6.568632368213271, "velocity"=0.2949641286481167, "acceleration"=0.09170049452982382, "pose"={"Translation2d"={"x"=4.43925506382969, "y"=7.356112426601046}, "Rotation2d"={"Theta"=-0.8329653207785563}}, "curvature"=-7.117736713801189}, {"t"=6.599844003444989, "velocity"=0.2978262510339498, "acceleration"=0.19436465441653678, "pose"={"Translation2d"={"x"=4.445250087048047, "y"=7.349066839277097}, "Rotation2d"={"Theta"=-0.8984558337431857}}, "curvature"=-7.020717906536788}, {"t"=6.630862316881653, "velocity"=0.3038551148056507, "acceleration"=0.29775030464725916, "pose"={"Translation2d"={"x"=4.450821733405006, "y"=7.341581188558189}, "Rotation2d"={"Theta"=-0.9631283452570845}}, "curvature"=-6.822334266969233}, {"t"=6.661507330894593, "velocity"=0.31297967706392316, "acceleration"=0.40207825036753225, "pose"={"Translation2d"={"x"=4.455968445233568, "y"=7.333653933868523}, "Rotation2d"={"Theta"=-1.0263282697065546}}, "curvature"=-6.536621755734763}, {"t"=6.691626862860313, "velocity"=0.3250900857785891, "acceleration"=0.5069727477723713, "pose"={"Translation2d"={"x"=4.460689621994987, "y"=7.32528453392471}, "Rotation2d"={"Theta"=-1.087488147579063}}, "curvature"=-6.182184923707348}, {"t"=6.721102904086689, "velocity"=0.3400336353925766, "acceleration"=0.611399064002761, "pose"={"Translation2d"={"x"=4.464985595149651, "y"=7.316473420438601}, "Rotation2d"={"Theta"=-1.1461488074139534}}, "curvature"=-5.77962728218252}, {"t"=6.749854018030981, "velocity"=0.35761203954715337, "acceleration"=0.7136909748896774, "pose"={"Translation2d"={"x"=4.46885760302794, "y"=7.307221971820122}, "Rotation2d"={"Theta"=-1.2019682666495493}}, "curvature"=-5.349154849994294}, {"t"=6.777834181656839, "velocity"=0.37758122980286485, "acceleration"=0.8116732069943011, "pose"={"Translation2d"={"x"=4.472307765701101, "y"=7.297532486880103}, "Rotation2d"={"Theta"=-1.254719563749324}}, "curvature"=-4.908764457929909}, {"t"=6.805028981536052, "velocity"=0.3996545202343935, "acceleration"=0.9028671117691384, "pose"={"Translation2d"={"x"=4.475339059852111, "y"=7.287408158533106}, "Rotation2d"={"Theta"=-1.3042802230553214}}, "curvature"=-4.473180516322608}, {"t"=6.831450240656345, "velocity"=0.423509406145637, "acceleration"=0.9847508747674881, "pose"={"Translation2d"={"x"=4.477955293646552, "y"=7.276853047500262}, "Rotation2d"={"Theta"=-1.3506165973360953}}, "curvature"=-4.053489703016462}, {"t"=6.857130057884056, "velocity"=0.4487976286244948, "acceleration"=1.0840978528150274, "pose"={"Translation2d"={"x"=4.480161081603476, "y"=7.265872056012099}, "Rotation2d"={"Theta"=-1.3937660908844118}}, "curvature"=-3.6572987095129776}, {"t"=6.906415424080401, "velocity"=0.5022277882931547, "acceleration"=1.1681738456180772, "pose"={"Translation2d"={"x"=4.48336365907354, "y"=7.242656090355901}, "Rotation2d"={"Theta"=-1.4709054934935915}}, "curvature"=-2.951411863769849}, {"t"=6.9534146874062905, "velocity"=0.5571310984737756, "acceleration"=1.193511382535945, "pose"={"Translation2d"={"x"=4.48499888057713, "y"=7.21781531030428}, "Rotation2d"={"Theta"=-1.5367982374777283}}, "curvature"=-2.3671059273267914}, {"t"=6.998610709889867, "velocity"=0.6110730657532749, "acceleration"=1.167228878425908, "pose"={"Translation2d"={"x"=4.48513012782019, "y"=7.191416545728572}, "Rotation2d"={"Theta"=-1.5927777102801355}}, "curvature"=-1.8952861433421067}, {"t"=7.0424478424442185, "velocity"=0.6622410328180989, "acceleration"=1.1031072318105943, "pose"={"Translation2d"={"x"=4.483831271767576, "y"=7.163537566122281}, "Rotation2d"={"Theta"=-1.6401769535401651}}, "curvature"=-1.5187654555632588}, {"t"=7.085299075903088, "velocity"=0.7095105383385827, "acceleration"=0.9684377738130721, "pose"={"Translation2d"={"x"=4.481185868510851, "y"=7.134266239091687}, "Rotation2d"={"Theta"=-1.680211297171634}}, "curvature"=-1.2191901359084476}, {"t"=7.169232040012571, "velocity"=0.790794391250303, "acceleration"=0.7862293281400811, "pose"={"Translation2d"={"x"=4.472233245591629, "y"=7.071943454690177}, "Rotation2d"={"Theta"=-1.7422278435917522}}, "curvature"=-0.7877885280324147}, {"t"=7.251717497665008, "velocity"=0.8556468772017057, "acceleration"=0.6443002943750661, "pose"={"Translation2d"={"x"=4.459103853305386, "y"=7.0053211182726045}, "Rotation2d"={"Theta"=-1.785308378900926}}, "curvature"=-0.5023790527257399}, {"t"=7.333169771733416, "velocity"=0.9081266013614995, "acceleration"=0.5623075046520477, "pose"={"Translation2d"={"x"=4.4427327834611825, "y"=6.935379868790441}, "Rotation2d"={"Theta"=-1.813745214747585}}, "curvature"=-0.3012612639388497}, {"t"=7.41328161180343, "velocity"=0.9531740902443532, "acceleration"=0.5488855969790963, "pose"={"Translation2d"={"x"=4.4241328932037085, "y"=6.863181130097338}, "Rotation2d"={"Theta"=-1.8302042982477884}}, "curvature"=-0.14628975216743031}, {"t"=7.491221325535914, "velocity"=0.9959540765447876, "acceleration"=-0.45125036796996526, "pose"={"Translation2d"={"x"=4.404369072782734, "y"=6.789840182648404}, "Rotation2d"={"Theta"=-1.8361458971072677}}, "curvature"=-0.012097016067171314}, {"t"=7.568872140041282, "velocity"=0.9609141179260725, "acceleration"=-0.5647024525910581, "pose"={"Translation2d"={"x"=4.384532513322541, "y"=6.716499235199469}, "Rotation2d"={"Theta"=-1.8320649407218288}}, "curvature"=0.12112540777990023}, {"t"=7.648374940406329, "velocity"=0.9160186915720734, "acceleration"=-0.6426968844949578, "pose"={"Translation2d"={"x"=4.365714974591368, "y"=6.644300496506366}, "Rotation2d"={"Theta"=-1.8175711668267878}}, "curvature"=0.27300978311453855}, {"t"=7.7291731327763475, "velocity"=0.8640899450630382, "acceleration"=-0.7840912084570016, "pose"={"Translation2d"={"x"=4.348983052770848, "y"=6.574359247024203}, "Rotation2d"={"Theta"=-1.7913197948653747}}, "curvature"=0.4683737482570857}, {"t"=7.810902047747827, "velocity"=0.8000070213571715, "acceleration"=-0.9717670823993614, "pose"={"Translation2d"={"x"=4.335352448225446, "y"=6.507736910606631}, "Rotation2d"={"Theta"=-1.750780406494041}}, "curvature"=0.7444248447082671}, {"t"=7.89390622691947, "velocity"=0.7193462923365892, "acceleration"=-1.1525167861686512, "pose"={"Translation2d"={"x"=4.325762233271908, "y"=6.4454141262051206}, "Rotation2d"={"Theta"=-1.6918170448995062}}, "curvature"=1.1618035078482665}, {"t"=7.979491291568851, "velocity"=0.6207080686828482, "acceleration"=-1.2279138106159257, "pose"={"Translation2d"={"x"=4.321049119948684, "y"=6.3882638195682375}, "Rotation2d"={"Theta"=-1.6080938154691222}}, "curvature"=1.819642710916439}, {"t"=8.023982023933382, "velocity"=0.5660772839680233, "acceleration"=-1.213987143459038, "pose"={"Translation2d"={"x"=4.32074862723075, "y"=6.361865054992528}, "Rotation2d"={"Theta"=-1.554229183834945}}, "curvature"=2.282635502335119}, {"t"=8.070204152701344, "velocity"=0.5099642139004098, "acceleration"=-1.1390484102972946, "pose"={"Translation2d"={"x"=4.321921727785386, "y"=6.337024274940908}, "Rotation2d"={"Theta"=-1.4905873873528683}}, "curvature"=2.8614621422727504}, {"t"=8.118660432929483, "velocity"=0.45477016493762756, "acceleration"=-1.0439844750065996, "pose"={"Translation2d"={"x"=4.32463276290521, "y"=6.31380830928471}, "Rotation2d"={"Theta"=-1.415749206631394}}, "curvature"=3.5701589836797614}, {"t"=8.143916319635684, "velocity"=0.42840341131382703, "acceleration"=-0.9632744975641985, "pose"={"Translation2d"={"x"=4.326582065968441, "y"=6.302827317796546}, "Rotation2d"={"Theta"=-1.3737223202829167}}, "curvature"=3.973165143670482}, {"t"=8.169919428646885, "velocity"=0.4033552795459559, "acceleration"=-0.8720074406733708, "pose"={"Translation2d"={"x"=4.3289348515722175, "y"=6.292272206763702}, "Rotation2d"={"Theta"=-1.328453402042927}}, "curvature"=4.404817963130555}, {"t"=8.19671230377379, "velocity"=0.3799916930782627, "acceleration"=-0.7728544180566954, "pose"={"Translation2d"={"x"=4.331695874175318, "y"=6.282147878416706}, "Rotation2d"={"Theta"=-1.2798699246501777}}, "curvature"=4.858736136815974}, {"t"=8.224319123226767, "velocity"=0.35865564069553557, "acceleration"=-0.6685443626921248, "pose"={"Translation2d"={"x"=4.334869086325574, "y"=6.272458393476687}, "Rotation2d"={"Theta"=-1.2279647766292976}}, "curvature"=5.324925338385862}, {"t"=8.252739248295114, "velocity"=0.3396555262940866, "acceleration"=-0.5615677589366793, "pose"={"Translation2d"={"x"=4.3384576135307515, "y"=6.263206944858208}, "Rotation2d"={"Theta"=-1.1728156577162963}}, "curvature"=5.789376201433284}, {"t"=8.281940952895548, "velocity"=0.3232567904844901, "acceleration"=-0.45392550811035604, "pose"={"Translation2d"={"x"=4.342463729129415, "y"=6.2543958313721}, "Rotation2d"={"Theta"=-1.1146035916342591}}, "curvature"=6.2341343733371914}, {"t"=8.311856306790474, "velocity"=0.3096774482674344, "acceleration"=-0.34696015155136106, "pose"={"Translation2d"={"x"=4.346888829161787, "y"=6.246026431428286}, "Rotation2d"={"Theta"=-1.0536275630080953}}, "curvature"=6.63807860036062}, {"t"=8.342378391588255, "velocity"=0.299087501100333, "acceleration"=-0.24128875012029047, "pose"={"Translation2d"={"x"=4.351733407240634, "y"=6.238099176738619}, "Rotation2d"={"Theta"=-0.9903117021356771}}, "curvature"=6.978554094160373}, {"t"=8.373362001111014, "velocity"=0.2916115046843714, "acceleration"=-0.13683731223853002, "pose"={"Translation2d"={"x"=4.356997029422121, "y"=6.230613526019712}, "Rotation2d"={"Theta"=-0.9252015770462301}}, "curvature"=7.233804284983293}, {"t"=8.404628601498835, "velocity"=0.2873330671244657, "acceleration"=-0.0329610042221216, "pose"={"Translation2d"={"x"=4.362678309076686, "y"=6.223567938695764}, "Rotation2d"={"Theta"=-0.858947336438271}}, "curvature"=7.385857232966142}, {"t"=8.435975588473887, "velocity"=0.28629983895443023, "acceleration"=0.07137487239675654, "pose"={"Translation2d"={"x"=4.36877488175991, "y"=6.216959848601399}, "Rotation2d"={"Theta"=-0.7922736994181268}}, "curvature"=7.4232587686803}, {"t"=8.467188931383573, "velocity"=0.2885276873216852, "acceleration"=0.17738135493703838, "pose"={"Translation2d"={"x"=4.375283380083379, "y"=6.210785637684495}, "Rotation2d"={"Theta"=-0.7259396414706673}}, "curvature"=7.342947416348255}, {"t"=8.49805743642295, "velocity"=0.2940031845704507, "acceleration"=0.2862274360275855, "pose"={"Translation2d"={"x"=4.382199408585557, "y"=6.205040609709009}, "Rotation2d"={"Theta"=-0.6606931857136173}}, "curvature"=7.150733890724849}, {"t"=8.528386421829314, "velocity"=0.30268417230063227, "acceleration"=0.3988427287997138, "pose"={"Translation2d"={"x"=4.389517518602659, "y"=6.199718963957817}, "Rotation2d"={"Theta"=-0.5972280125257339}}, "curvature"=6.8602464870692}, {"t"=8.558008758144027, "velocity"=0.31449882574981547, "acceleration"=0.5157652082661012, "pose"={"Translation2d"={"x"=4.39723118313951, "y"=6.1948137689355445}, "Rotation2d"={"Theta"=-0.5361481172995023}}, "curvature"=6.4906633425954885}, {"t"=8.586791919034814, "velocity"=0.32934417872120925, "acceleration"=0.6370555206593937, "pose"={"Translation2d"={"x"=4.405332771740426, "y"=6.1903169360713886}, "Rotation2d"={"Theta"=-0.47794467568292925}}, "curvature"=6.063866284442087}, {"t"=8.614640634674986, "velocity"=0.3470853567630544, "acceleration"=0.762294606301549, "pose"={"Translation2d"={"x"=4.413813525360063, "y"=6.186219193421963}, "Rotation2d"={"Theta"=-0.42298643498376026}}, "curvature"=5.601702319766141}, {"t"=8.641495606692553, "velocity"=0.36755675708442503, "acceleration"=0.8906732669703521, "pose"={"Translation2d"={"x"=4.422663531234306, "y"=6.182510059374114}, "Rotation2d"={"Theta"=-0.37152232606286834}}, "curvature"=5.123857637458907}, {"t"=8.6673292997755, "velocity"=0.3905661369005225, "acceleration"=1.0211712999910656, "pose"={"Translation2d"={"x"=4.431871697751131, "y"=6.179177816347768}, "Rotation2d"={"Theta"=-0.3236932778807256}}, "curvature"=4.646563802534958}, {"t"=8.692140008791045, "velocity"=0.4159021208796266, "acceleration"=1.21985317023459, "pose"={"Translation2d"={"x"=4.441425729321469, "y"=6.17620948449875}, "Rotation2d"={"Theta"=-0.2795496156304768}}, "curvature"=4.1820999036195605}, {"t"=8.738686024996154, "velocity"=0.4726814263092206, "acceleration"=1.4858556710690907, "pose"={"Translation2d"={"x"=4.461516034606399, "y"=6.171306165852511}, "Rotation2d"={"Theta"=-0.20218442338018275}}, "curvature"=3.3220368096181314}, {"t"=8.781507525991874, "velocity"=0.5363079964074019, "acceleration"=0.03687477342119676, "pose"={"Translation2d"={"x"=4.482811047928713, "y"=6.167670020107663}, "Rotation2d"={"Theta"=-0.1387458343095483}}, "curvature"=2.57463247596816}, {"t"=8.823395376425081, "velocity"=0.5378526014012274, "acceleration"=-1.4999999999999993, "pose"={"Translation2d"={"x"=4.505166498230942, "y"=6.165149084692138}, "Rotation2d"={"Theta"=-0.08822539249239807}}, "curvature"=1.9372423652832413}, {"t"=8.925941341069555, "velocity"=0.38403365443451604, "acceleration"=-1.5, "pose"={"Translation2d"={"x"=4.5523724412666065, "y"=6.162730549282688}, "Rotation2d"={"Theta"=-0.022237140076903836}}, "curvature"=0.9060261366102136}, {"t"=9.181963777359233, "velocity"=0.0, "acceleration"=-1.5, "pose"={"Translation2d"={"x"=4.601531700288179, "y"=6.162365296803663}, "Rotation2d"={"Theta"=2.2425669336754695e-14}}, "curvature"=4.5298163886599506e-14}], 6 "Reverse Path?":bool)   [LabVIEW 2019]
uses:
  AutonBuilder/Typedef/Data Point.ctl
  <vilib>/Rock Robotics/WPI/ThirdParty/WPILib Extensions/Trajectory/Typedef/Trajectory State.ctl
  <vilib>/Rock Robotics/WPI/ThirdParty/WPILib Extensions/Geometry/Typedef/Pose2d.ctl
  <vilib>/Rock Robotics/WPI/ThirdParty/WPILib Extensions/Geometry/Typedef/Translation2d.ctl
  <vilib>/Rock Robotics/WPI/ThirdParty/WPILib Extensions/Geometry/Typedef/Rotation2d.ctl
panel:
  out "Total Time (s)":dbl=9.181963777359233
  out "Graph":cluster{dbl[], dbl[]}[](graph)=[{[2.848, 3.548, 3.548, 2.848, 2.848], [7.62, 7.62, 7.0200000000000005, 7.0200000000000005, 7.62]}, {[3.048, 6.688056195965419, 3.7631959654178675, 4.191678674351586, 4.601531700288184, 5.141792507204611], [7.32, 5.843945205479453, 6.124904109589042, 7.417315068493152, 6.162365296803654, 7.417315068493152]}, {array[201 elements], array[201 elements]}, {array[201 elements], array[201 elements]}, {array[201 elements], array[201 elements]}]
  in  "Data Points":T5[](array[typedef])=[{"X"=3.048, "Y"=7.32, "Theta"=0.0, "Speed %"=0.0, "Disabled?"=FALSE}, {"X"=6.688056195965419, "Y"=5.843945205479453, "Theta"=0.0, "Speed %"=0.0, "Disabled?"=TRUE}, {"X"=3.7631959654178675, "Y"=6.124904109589042, "Theta"=0.0, "Speed %"=0.0, "Disabled?"=FALSE}, {"X"=4.191678674351586, "Y"=7.417315068493152, "Theta"=0.0, "Speed %"=0.0, "Disabled?"=FALSE}, {"X"=4.601531700288184, "Y"=6.162365296803654, "Theta"=0.0, "Speed %"=0.0, "Disabled?"=FALSE}, {"X"=5.141792507204611, "Y"=7.417315068493152, "Theta"=0.0, "Speed %"=0.0, "Disabled?"=TRUE}]
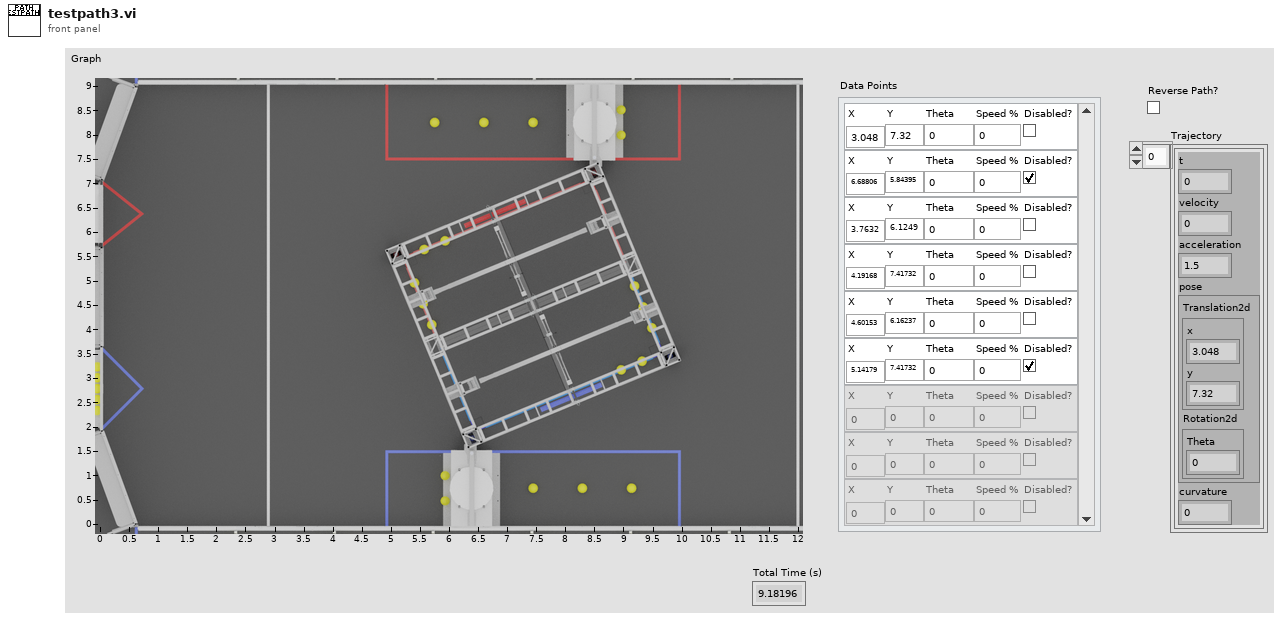
[diagram p1: front panel]
types:
  T1 = typedef "Trajectory State.ctl" = cluster{"t":dbl, "velocity":dbl, "acceleration":dbl, "pose":T2, "curvature":dbl}
  T2 = typedef "Pose2d.ctl" = cluster{"Translation2d":T3, "Rotation2d":T4}
  T3 = typedef "Translation2d.ctl" = cluster{"x":dbl, "y":dbl}
  T4 = typedef "Rotation2d.ctl" = cluster{"Theta":dbl}
  T5 = typedef "Data Point.ctl" = cluster{"X":dbl, "Y":dbl, "Theta":dbl, "Speed %":dbl, "Disabled?":bool}
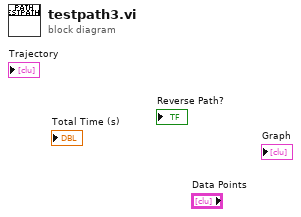
[diagram p0: block diagram]
diagram:
